vi "Main.vi"() -> ()   [LabVIEW 2021]
uses:
  <vilib>/Platform/TimedLoop/XDataNode/timing_clust.ctl
  <vilib>/Platform/TimedLoop/XDataNode/nitl_modes.ctl
  <vilib>/Platform/TimedLoop/XDataNode/wakeup.ctl
  <vilib>/myRIO/Instrument Drivers/Onboard IO/PWM/typedefs/PWM Reference.ctl
  <vilib>/myRIO/Common/Instrument Driver Framework/Utilities/typedefs/myRIO Generic Hardware Reference.ctl
  <vilib>/myRIO/Common/Instrument Driver Framework/Utilities/typedefs/Hardware Version Enum.ctl
  <vilib>/myRIO/Common/Instrument Driver Framework/Utilities/typedefs/myRIO v1.0 Reference.ctl
  <vilib>/myRIO/Common/Instrument Driver Framework/Utilities/typedefs/Generic FPGA Reference.ctl
  <vilib>/myRIO/Common/Instrument Driver Framework/myRIO v1.0/PWM/typedefs/PWM Channels Enum.ctl
  <vilib>/myRIO/Instrument Drivers/Onboard IO/PWM/typedefs/PWM Configuration.ctl
  <vilib>/userDefined/High Color/nirio_resource_hc.ctl
  <vilib>/myRIO/Common/Instrument Driver Framework/Utilities/vis/Is FPGA Ref Available.vi
  <vilib>/myRIO/Common/Instrument Driver Framework/myRIO v1.0/PWM/vis/myRIO v1.1 Open PWM.vi
  <vilib>/myRIO/Instrument Drivers/Onboard IO/PWM/vis/Set Duty Cycle and Frequency.vi
  <vilib>/myRIO/Common/Instrument Driver Framework/Utilities/vis/Validate Channels.vi
  <vilib>/myRIO/Common/Instrument Driver Framework/myRIO v1.0/PWM/vis/myRIO v1.0 Reserve PWM.vi
  <vilib>/myRIO/Common/Instrument Driver Framework/myRIO v1.0/UART/vis/myRIO v1.0 Close UART.vi
  <vilib>/myRIO/Common/Instrument Driver Framework/myRIO v1.0/PWM/vis/myRIO v1.0 Build MUX Configuration PWM.vi
  <vilib>/myRIO/Common/Instrument Driver Framework/myRIO v1.0/Resource Manager/vis/myRIO v1.0 Reserve Channel List.vi
  <vilib>/myRIO/Common/Instrument Driver Framework/myRIO v1.0/Resource Manager/vis/myRIO v1.0 Create Configuration List.vi
  <vilib>/myRIO/Common/Instrument Driver Framework/myRIO v1.0/Resource Manager/vis/myRIO v1.0 Reserve Channel.vi
  <vilib>/myRIO/Common/Instrument Driver Framework/myRIO v1.0/Resource Manager/vis/myRIO v1.0 Unreserve Channel.vi
  <vilib>/myRIO/Common/Instrument Driver Framework/myRIO v1.0/Resource Manager/vis/myRIO v1.0 Build Mutex Name.vi
  <vilib>/Utility/VariantDataType/GetNumericInfo.vi
  <vilib>/Utility/error.llb/Error Cluster From Error Code.vi
  <vilib>/myRIO/Common/Instrument Driver Framework/myRIO v1.0/myRIO v1.1 Open.vi
  <vilib>/myRIO/Common/Instrument Driver Framework/Utilities/vis/IO Manager.vi
  <vilib>/myRIO/Common/Instrument Driver Framework/Utilities/vis/Configuration Manager.vi
  <vilib>/myRIO/Common/Instrument Driver Framework/myRIO v1.0/Resource Manager/vis/myRIO v1.0 Configure IO.vi
  <vilib>/myRIO/Common/Instrument Driver Framework/myRIO v1.0/myRIO v1.0 Close.vi
  <vilib>/myRIO/Common/Instrument Driver Framework/myRIO v1.0/PWM/vis/myRIO v1.0 Write PWM.vi
  <vilib>/myRIO/Common/Instrument Driver Framework/Utilities/vis/FPGA Ref Manager.vi
  <vilib>/myRIO/Common/Instrument Driver Framework/myRIO v1.0/myRIO v1.0 Reset FPGA.vi
  <vilib>/myRIO/Common/Instrument Driver Framework/myRIO v1.0/IRQ/vis/myRIO v1.0 IRQ Info FGV.vi
  <vilib>/myRIO/Common/Instrument Driver Framework/myRIO v1.0/IRQ/vis/myRIO v1.0 Timer IRQ Info FGV.vi
  <vilib>/myRIO/Common/Instrument Driver Framework/myRIO v1.0/IRQ/vis/myRIO v1.0 ISR Agent.vi
  <vilib>/myRIO/Instrument Drivers/Utilities/vis/Reset Index.vi
  <vilib>/myRIO/Common/Instrument Driver Framework/myRIO v1.0/Resource Manager/vis/myRIO v1.0 Block Write Resource Manager.vi
  <vilib>/Platform/TimedLoop/XDataNode/XDataNode.xnode
  <vilib>/myRIO/Express VI/Onboard IO/PWM/PWM Express VI.xnode
  <vilib>/myRIO/Instrument Drivers/Onboard IO/PWM/vis/myRIO PWM Open.xnode
  <vilib>/myRIO/Common/Instrument Driver Framework/myRIO v1.0/Encoder/typedefs/Encoder Signal Mode.ctl
  <vilib>/myRIO/Common/Instrument Driver Framework/myRIO v1.0/Encoder/typedefs/Encoder Channels Enum.ctl
  <vilib>/myRIO/Instrument Drivers/Onboard IO/Encoder/typedefs/Encoder Reference.ctl
  <vilib>/myRIO/Instrument Drivers/Onboard IO/Encoder/Encoder.lvlib
  <vilib>/myRIO/Instrument Drivers/Onboard IO/Encoder/vis/Read.vi
  <vilib>/myRIO/Common/Instrument Driver Framework/myRIO v1.0/Encoder/typedefs/Encoder Configuration v1.0.ctl
  <vilib>/myRIO/Common/Instrument Driver Framework/myRIO v1.0/Encoder/vis/myRIO v1.1 Open Encoder.vi
  <vilib>/myRIO/Common/Instrument Driver Framework/myRIO v1.0/Encoder/vis/myRIO v1.0 Configure Encoder.vi
  <vilib>/myRIO/Instrument Drivers/Onboard IO/Encoder/vis/myRIO Encoder Open.xnode
  <vilib>/myRIO/Express VI/Onboard IO/Encoder/Encoder Express VI.xnode
  <vilib>/myRIO/Instrument Drivers/Onboard IO/PWM/PWM.lvlib
  <vilib>/myRIO/Instrument Drivers/Utilities/Utilities.lvlib
  <vilib>/Platform/TimedLoop/XDataNode/XDNodeRunTimeDep.lvlib
panel:
  out "Last Measure":dbl
  in  "Limit switch":bool
  in  "stop":bool
  in  "Measure":bool
  in  "X":dbl(slide) scale=0.0..200.0
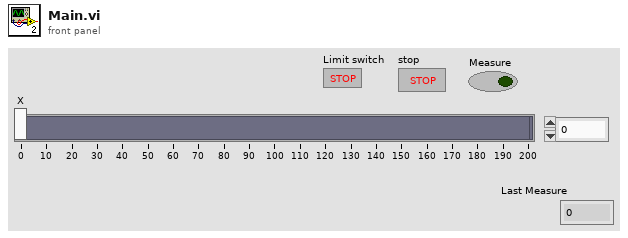
[diagram p1: front panel]
types:
  T1 = typedef "Encoder.lvlib/Encoder Reference.ctl" = cluster{"myRIO Reference":T2, "Encoder Channels Enum":T6}
  T2 = typedef "myRIO Generic Hardware Reference.ctl" = cluster{"myRIO Model":T3, "myRIO Hardware Reference":T4}
  T3 = typedef "Hardware Version Enum.ctl" = enum16{"Unknown", "myRIO-1900", "myRIO-1950", "roboRIO", "NI ELVIS RIO CM", "ELVIS III"}
  T4 = typedef "myRIO v1.0 Reference.ctl" = cluster{"Generic FPGA Reference":T5, "Allow multiple opens":bool}
  T5 = typedef "Generic FPGA Reference.ctl" = refnum<k20>
  T6 = typedef "Encoder Channels Enum.ctl" = enum16{"Not Connected", "C/ENC0", "C/ENC1", "A/ENC", "A/ENC0", "A/ENC1", "A/ENC2", "A/ENC3", "A/ENC4", "A/ENC5", "A/ENC6", "A/ENC7", "A/ENC8", "A/ENC9", "B/ENC", "B/ENC0", "B/ENC1", "B/ENC2", "B/ENC3", "B/ENC4", "B/ENC5", "B/ENC6", "B/ENC7", "B/ENC8", "B/ENC9", "DIO/ENC0", "DIO/ENC1", "DIO/ENC2", "DIO/ENC3", "DIO/ENC4"}
  T7 = typedef "Encoder Signal Mode.ctl" = enum16{"Quadrature phase signal", "Step and direction signal"}
  T8 = typedef "nirio_resource_hc.ctl" = tag
  T9 = typedef "XDNodeRunTimeDep.lvlib/timing_clust.ctl" = cluster{"Expected End [f-1]":u64, "Actual End [f-1]":u64, "Finished Late? [f-1]":bool, "Expected End [i-1]":u64, "Actual End [i-1]":u64, "Finished Late? [i-1]":bool, "Expected Start [i]":u64, "Actual Start [i]":u64, "Expected Start [f]":u64, "Actual Start [f]":u64, "Source Name":string, "Structure Name":string, "Period":i64, "Deadline":i64, "Offset":i64, "Start":i64, "Priority":i32, "Timeout":i32, "Mode":T10, "Wakeup Reason":T11, "Error":errorcluster, "Source Type":string, "Secondary Source Type":string, "Global End Time":u64, "Global Start Time":u64, "Frame Duration":u64, "Iteration Duration":u64, "Assigned CPU":i32, "I/O Scan Engine Mode":u32}
  T10 = typedef "XDNodeRunTimeDep.lvlib/nitl_modes.ctl" = enum32{"No Change", "Process missed periods, maintain original phase", "Discard missed periods, maintain original phase", "Process missed periods, ignore original phase", "Discard missed periods, ignore original phase"}
  T11 = typedef "XDNodeRunTimeDep.lvlib/wakeup.ctl" = enum32{"Normal", "Aborted", "Asynchronous wakeup", "Timing source error", "Timed loop error", "Timeout"}
  T12 = enum8{"Enabled", "Disabled", "Disabled and Grayed Out"}
  T13 = typedef "PWM.lvlib/PWM Reference.ctl" = cluster{"myRIO Reference":T2, "PWM Channels Enum":T14, "PWM Configuration":T15}
  T14 = typedef "PWM Channels Enum.ctl" = enum16{"Not Connected", "C/PWM0", "C/PWM1", "A/PWM0", "A/PWM1", "A/PWM2", "A/PWM3", "A/PWM4", "A/PWM5", "A/PWM6", "A/PWM7", "A/PWM8", "A/PWM9", "A/PWM10", "A/PWM11", "A/PWM12", "A/PWM13", "A/PWM14", "A/PWM15", "A/PWM16", "A/PWM17", "A/PWM18", "A/PWM19", "B/PWM0", "B/PWM1", "B/PWM2", "B/PWM3", "B/PWM4", "B/PWM5", "B/PWM6", "B/PWM7", "B/PWM8", "B/PWM9", "B/PWM10", "B/PWM11", "B/PWM12", "B/PWM13", "B/PWM14", "B/PWM15", "B/PWM16", "B/PWM17", "B/PWM18", "B/PWM19", "PWM/PWM0", "PWM/PWM1", "PWM/PWM2", "PWM/PWM3", "PWM/PWM4", "PWM/PWM5", "PWM/PWM6", "PWM/PWM7", "PWM/PWM8", "PWM/PWM9"}
  T15 = typedef "PWM.lvlib/PWM Configuration.ctl" = cluster{"Frequency":dbl, "Duty Cycle":dbl}
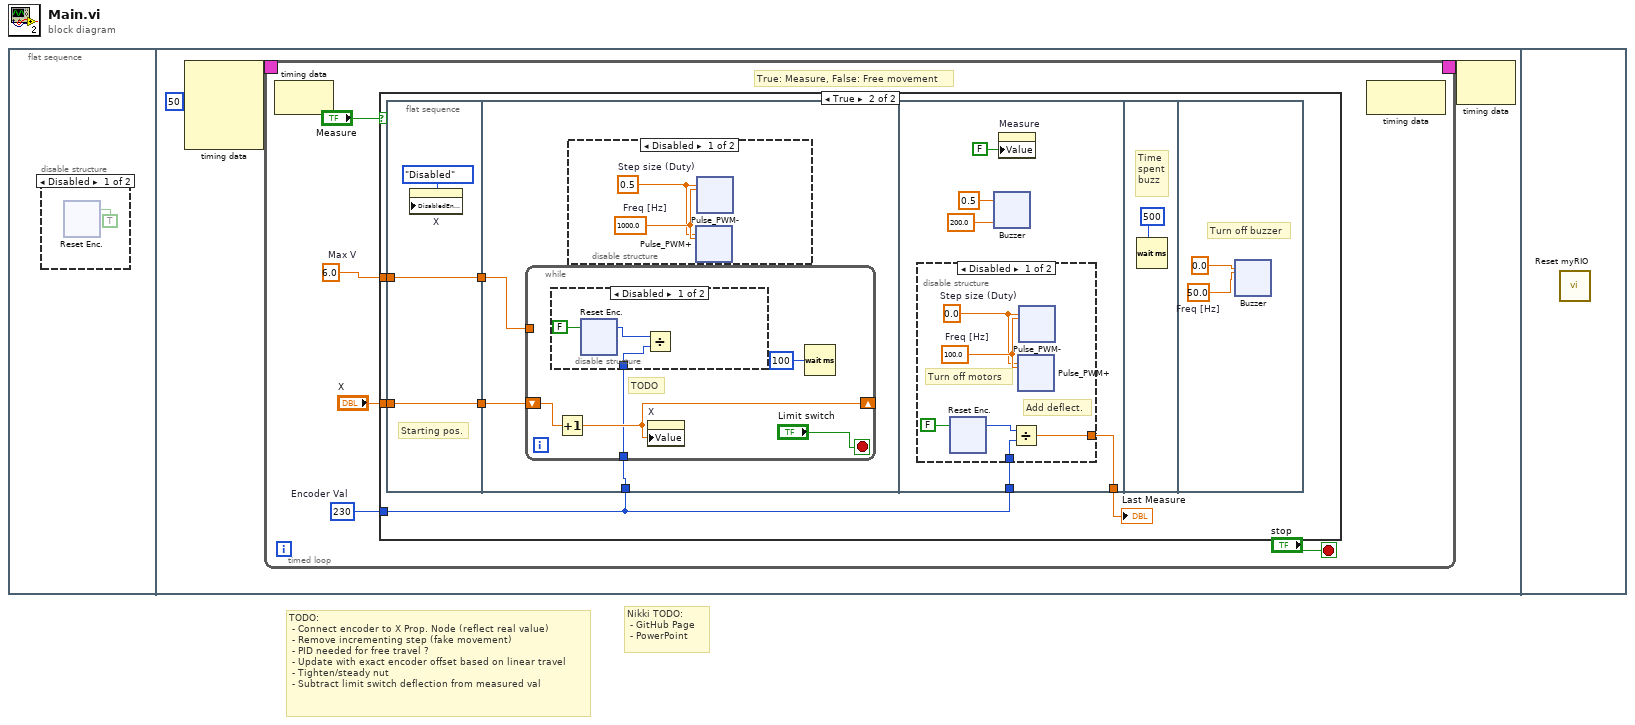
[diagram p0: block diagram]
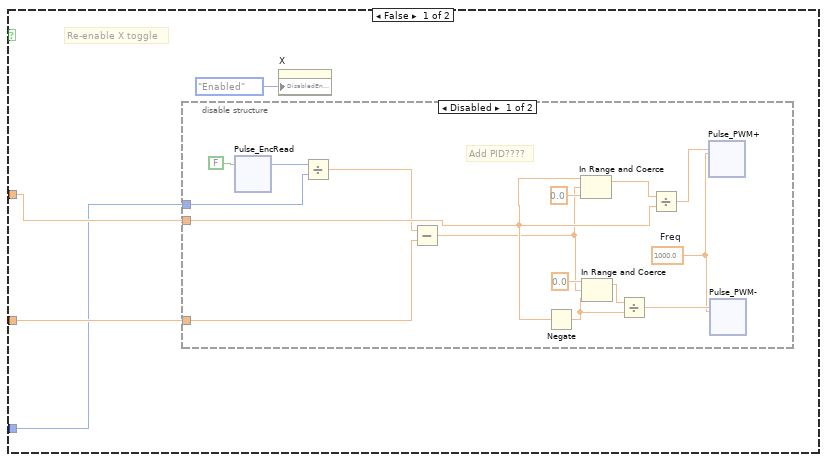
[diagram p3: hidden frame]
diagram:
  # "Nikki TODO:\n - GitHub Page \n - PowerPoint"
  # "TODO: \n - Connect encoder to X Prop. Node (reflect real value)\n - Remove incrementing step (fake movement)\n - PID needed for free travel ? \n - Update with exact encoder offset based on linear travel\n - Tighten/steady nut  \n - Subtract limit switch deflection from measured val"
  n1 = flat-sequence {
    frame #0 {
      n2 = disable-structure shown="Disabled" {
        frame Disabled {
          n3 = xnode "Reset Enc."("Reset Counter"=TRUE) -> ()  [unwired: 1 in, 4 out]
        }
        frame Enabled {
        }
      }
    }
    frame #1 {
      n4 = node-c288(i64 50 ("Period")) -> (w50:T9)  [unwired: 3 in]
      n5 = timed-loop {
        timing: w50 -> [_]
        timing-out: [_] -> w49
        stop <- "stop" stop-if-true
        w51 = 230  # Encoder Val
        w52 = 6.0  # Max V
        # "True: Measure, False: Free movement"
        n6 = node-c288() -> ()  [unwired: 1 in, 1 out]
        n7 = case shown="True" "Measure" {
          tunnel: "X" -> [w60 w198]
          tunnel: w52 -> [w59 w197]
          tunnel: w51 -> [w58 w194]
          frame False {
            # "Re-enable X toggle"
            n8 = disable-structure shown="Disabled" {
              disable-tunnel: w60 -> [w76 _]
              disable-tunnel: w59 -> [w75 _]
              disable-tunnel: w58 -> [w62 _]
              frame Disabled {
                w63 = 1000.0  # Freq
                # "Add PID????"
                n9 = xnode "Pulse_EncRead"("Reset Counter"=FALSE) -> ("Counter Value"=w73:i32)  [unwired: 1 in, 3 out]
                n10 = Divide(x=w73, y=w62) -> (x/y=w72:dbl)
                n11 = Subtract(x=w72, y=w76) -> (x-y=w64:dbl)
                n12 = Negate(x=w75) -> (-x=w65:dbl)
                n13 = In Range and Coerce(upper limit=w75, x=w64, lower limit=0.0) -> (coerced(x)=w71:dbl)  [unwired: 1 out]
                n14 = In Range and Coerce ("In Range and Coerce 2")(upper limit=0.0 ("lower limit 2"), x=w64, lower limit=w65) -> (coerced(x)=w68:dbl)  [unwired: 1 out]
                n15 = Divide ("Divide 3")(x=w68, y=w65) -> (x/y=w66:dbl)
                n16 = Divide ("Divide 2")(x=w71, y=w75) -> (x/y=w69:dbl)
                n17 = xnode "Pulse_PWM+"("Duty Cycle"=w69, "Frequency [Hz]"=w63) -> ()  [unwired: 1 in, 1 out]
                n18 = xnode "Pulse_PWM-"("Duty Cycle"=w66, "Frequency [Hz]"=w63) -> ()  [unwired: 1 in, 1 out]
              }
              frame Enabled {
              }
            }
            n19 = property on="X" class="Slide (strict)"("DisabledEnum"=T12."Enabled" ("Disabled")) -> ()  [unwired: 2 in, 2 out]
          }
          frame True {
            n20 = flat-sequence {
              tunnel: w197 -> [w200]
              tunnel: w198 -> [w201]
              tunnel: [w201] -> w196
              tunnel: [w200] -> w195
              tunnel: w196 -> [w204]
              tunnel: w195 -> [w203]
              tunnel: w194 -> [w202]
              tunnel: w194 -> [w332]
              tunnel: [w331] -> w193
              frame #0 {
                # "Starting pos."
                n21 = property on="X" class="Slide (strict)"("DisabledEnum"=T12."Disabled" ("Disabled")) -> ()  [unwired: 2 in, 2 out]
              }
              frame #1 {
                n22 = while {
                  tunnel: w203 -> [_]
                  shift-right: [w278] -> _
                  shift-left: w204 -> [w280]
                  tunnel: w202 -> [w277]
                  stop <- "Limit switch" stop-if-true
                  # "TODO"
                  n23 = disable-structure shown="Disabled" {
                    disable-tunnel: w277 -> [w283 _]
                    frame Disabled {
                      n24 = xnode "Reset Enc."("Reset Counter"=FALSE) -> ("Counter Value"=w284:i32)  [unwired: 1 in, 3 out]
                      n25 = Divide(x=w284, y=w283) -> ()  [unwired: 1 out]
                    }
                    frame Enabled {
                    }
                  }
                  n26 = Increment(x=w280) -> (x+1=w278:dbl)
                  n27 = property on="X" class="Slide (strict)"("Value"=w278) -> ()  [unwired: 2 in, 2 out]
                  n28 = Wait (ms)(milliseconds to wait=u32 100) -> ()  [unwired: 1 out]
                }
                n29 = disable-structure shown="Disabled" {
                  frame Disabled {
                    w205 = 0.5  # Step size (Duty)
                    w206 = 1000.0  # Freq [Hz]
                    n30 = xnode "Pulse_PWM+"("Duty Cycle"=w205, "Frequency [Hz]"=w206) -> ()  [unwired: 1 in, 1 out]
                    n31 = xnode "Pulse_PWM-"("Duty Cycle"=w205, "Frequency [Hz]"=w206) -> ()  [unwired: 1 in, 1 out]
                  }
                  frame Enabled {
                  }
                }
              }
              frame #2 {
                n32 = disable-structure shown="Disabled" {
                  disable-tunnel: w332 -> [w372 _]
                  disable-tunnel: [w371 _] -> w331
                  frame Disabled {
                    w375 = 0.0  # Step size (Duty)
                    w376 = 100.0  # Freq [Hz]
                    # "Add deflect."
                    # "Turn off motors"
                    n33 = xnode "Reset Enc."("Reset Counter"=FALSE) -> ("Counter Value"=w373:i32)  [unwired: 1 in, 3 out]
                    n34 = Divide(x=w373, y=w372) -> (x/y=w371:dbl)
                    n35 = xnode "Pulse_PWM+"("Duty Cycle"=w375, "Frequency [Hz]"=w376) -> ()  [unwired: 1 in, 1 out]
                    n36 = xnode "Pulse_PWM-"("Duty Cycle"=w375, "Frequency [Hz]"=w376) -> ()  [unwired: 1 in, 1 out]
                  }
                  frame Enabled {
                  }
                }
                n37 = xnode "Buzzer"("Duty Cycle"=0.5, "Frequency [Hz]"=200.0) -> ()  [unwired: 1 in, 1 out]
                n38 = property on="Measure" class="Bool (strict)"("Value"=FALSE ("State control")) -> ()  [unwired: 2 in, 2 out]
              }
              frame #3 {
                # "Time\nspent\nbuzz"
                n39 = Wait (ms)(milliseconds to wait=u32 500) -> ()  [unwired: 1 out]
              }
              frame #4 {
                w494 = 50.0  # Freq [Hz]
                # "Turn off buzzer"
                n40 = xnode "Buzzer"("Duty Cycle"=0.0, "Frequency [Hz]"=w494) -> ()  [unwired: 1 in, 1 out]
              }
            }
            "Last Measure" <- w193
          }
        }
        n41 = node-c288() -> ()  [unwired: 1 in, 1 out]
      }
      n42 = node-c288(w49) -> ()  [unwired: 1 out]
    }
    frame #2 {
      n43 = call <vilib>:"Reset myRIO.vi"() -> ()  [unwired: 11 in, 1 out]
    }
  }
